vi "Refresh Mulitlink XML.vi"(8 "error in":errorcluster, 9 "Chassis Name":string, 10 "Referencing Chassis":string[](array[string]), 11 "Cfg GM":refnum<class "Cfg Grandmaster.lvclass">) -> (0 "error out":errorcluster, 3 "Cfg GM":refnum<class "Cfg Grandmaster.lvclass">)   [LabVIEW 2012, in "Configuration Grandmaster.lvlib" / "Cfg Grandmaster.lvclass"]
uses:
  Cfg Grandmaster.lvclass
  Cfg Grandmaster.lvclass/Cfg Grandmaster.ctl
  Class FP Ctrls/FP Controls.lvclass
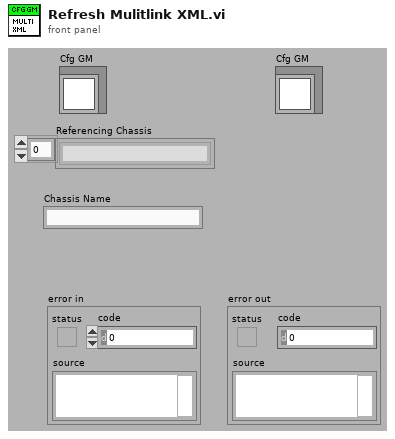
[diagram p1: front panel]
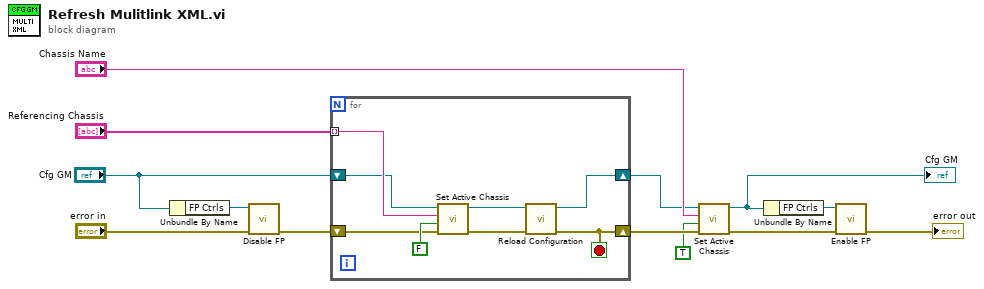
[diagram p0: block diagram]
diagram:
  n1 = Unbundle By Name("Cfg GM") -> ("FP Ctrls"=w3:refnum<class "FP Controls.lvclass">)
  n2 = call "Disable FP.vi"("error in (no error)"="error in", "FP Controls in"=w3) -> ("error out"=w11:errorcluster)  [unwired: 8 in, 1 out]
  n3 = for {
    tunnel: "Referencing Chassis" -> [w19] mode=indexing
    shift-right: [w17] -> w9
    shift-left: w11 -> [w20]
    shift-right: [w15] -> w5
    shift-left: "Cfg GM" -> [w14]
    stop <- w17 stop-if-true
    n4 = call "Set Active Chassis.vi"("error in (no error)"=w20, "Rfrsh GUI? (T)"=FALSE ("Rfrsh GUI?"), "Chassis Name"=w19, "Cfg Grandmaster in"=w14) -> ("error out"=w18:errorcluster, "Cfg Grandmaster out"=w16:refnum<class "Cfg Grandmaster.lvclass">)  [unwired: 6 in]
    n5 = call "Reload Configuration.vi"("error in (no error)"=w18, "Cfg Grandmaster in"=w16) -> ("error out"=w17:errorcluster, "Cfg Grandmaster out"=w15:refnum<class "Cfg Grandmaster.lvclass">)  [unwired: 8 in]
  }
  n6 = call "Set Active Chassis.vi"("error in (no error)"=w9, "Rfrsh GUI? (T)"=TRUE ("Rfrsh GUI?"), "Chassis Name"="Chassis Name", "Cfg Grandmaster in"=w5) -> ("error out"=w8:errorcluster, "Cfg Grandmaster out"=w1:refnum<class "Cfg Grandmaster.lvclass">)  [unwired: 6 in]
  "Cfg GM" <- w1
  n7 = Unbundle By Name(w1) -> ("FP Ctrls"=w2:refnum<class "FP Controls.lvclass">)
  n8 = call "Enable FP.vi"("error in (no error)"=w8, "FP Controls in"=w2) -> ("error out"=→"error out":errorcluster)  [unwired: 8 in, 1 out]
